vi "LoadTest.vi"() -> ()   [LabVIEW 2013]
uses:
  <vilib>/MDSplus/Library/MDSplus.lvlib
panel:
  out "I32 out":i32
  in  "Node Path/tag 3":string="\\proto_tree::TOP.NI_DAQ.DAQ_0.CHANNEL_0.CHAN_SETTING:ACTIVE"
  out "DBL out":dbl
  in  "Node Path/tag 2":string="\\proto_tree::TOP.NI_DAQ.DAQ_0.CHANNEL_0.CHAN_SETTING:VOLT_RANGE"
  out "String value out":string
  in  "Shot Number":i32=182
  in  "Tree name":string="proto_tree"
  in  "Node Path/tag 1":string="\\proto_tree::TOP.NI_DAQ.DAQ_0.CHANNEL_0.CHAN_SETTING:CHANNEL_NAME"
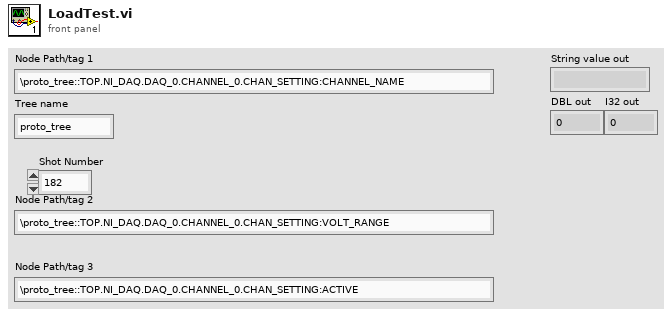
[diagram p1: front panel]
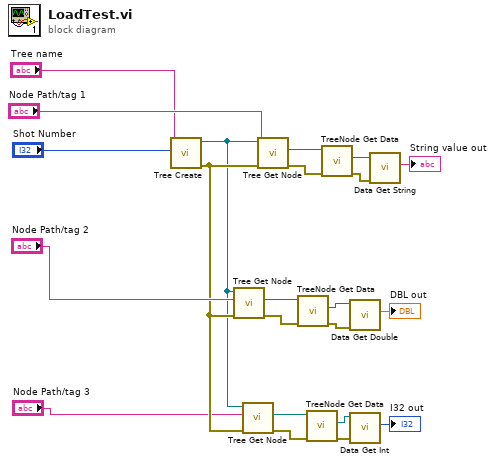
[diagram p0: block diagram]
diagram:
  n1 = call <vilib>:"Tree Create.vi"("Shot"="Shot Number", "Name"="Tree name") -> ("error out"=w6:errorcluster, "Tree DVR out"=w5:refnum<data-value>)  [unwired: 8 in]
  n2 = call <vilib>:"Tree Get Node.vi"("error in (no error)"=w6, "Path"="Node Path/tag 2", "Tree DVR in"=w5) -> ("error out"=w14:errorcluster, "Node out"=w13:refnum<data-value>)  [unwired: 6 in, 1 out]
  n3 = call <vilib>:"Tree Get Node.vi"("error in (no error)"=w6, "Path"="Node Path/tag 3", "Tree DVR in"=w5) -> ("error out"=w7:errorcluster, "Node out"=w8:refnum<data-value>)  [unwired: 6 in, 1 out]
  n4 = call <vilib>:"Tree Get Node.vi"("error in (no error)"=w6, "Path"="Node Path/tag 1", "Tree DVR in"=w5) -> ("error out"=w18:errorcluster, "Node out"=w19:refnum<data-value>)  [unwired: 6 in, 1 out]
  n5 = call <vilib>:"TreeNode Get Data.vi"("error in (no error)"=w14, "TreeNode DVR in"=w13) -> ("error out"=w11:errorcluster, "Data out"=w10:refnum<data-value>)  [unwired: 7 in, 1 out]
  n6 = call <vilib>:"TreeNode Get Data.vi"("error in (no error)"=w7, "TreeNode DVR in"=w8) -> ("error out"=w3:errorcluster, "Data out"=w2:refnum<data-value>)  [unwired: 7 in, 1 out]
  n7 = call <vilib>:"TreeNode Get Data.vi"("error in (no error)"=w18, "TreeNode DVR in"=w19) -> ("error out"=w17:errorcluster, "Data out"=w16:refnum<data-value>)  [unwired: 7 in, 1 out]
  n8 = call <vilib>:"Data Get Double.vi"("error in (no error)"=w11, "Data DVR in"=w10) -> ("DBL out"=→"DBL out":dbl)  [unwired: 7 in, 2 out]
  n9 = call <vilib>:"Data Get Int.vi"("error in (no error)"=w3, "Data DVR in"=w2) -> ("I32 out"=→"I32 out":i32)  [unwired: 7 in, 2 out]
  n10 = call <vilib>:"Data Get String.vi"("error in (no error)"=w17, "Data DVR in"=w16) -> ("String value out"=→"String value out":string)  [unwired: 7 in, 2 out]
